vi "BeginTest.vi"(8 "error in":errorcluster) -> (0 "error out":errorcluster)   [LabVIEW 2015]
doc: "Called before other user functions, this VI is expected to open initial I/O refnums, load in file data, and do all program initialization. Notice that the <B>error out</B> terminal is simply used for data flow. Wiring it to other structures or subVIs ensures that this VI runs first."
uses:
  <vilib>/Rock Robotics/WPI/DriverStation/WPI_DriverStationRobotMode2.ctl
  <vilib>/Rock Robotics/WPI/Joystick/WPI_JoystickDeviceEnum.ctl
  <vilib>/Rock Robotics/WPI/Solenoid/WPI_SolenoidChannel.ctl
  <vilib>/Rock Robotics/SystemInterfaces/DIO/FPGA_DIOChannel.ctl
  Robot Global Data.vi
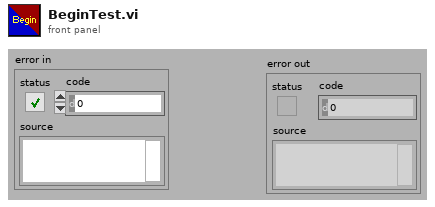
[diagram p1: front panel]
types:
  T1 = typedef "WPI_SolenoidChannel.ctl" = enum8{"Solenoid 0", "Solenoid 1", "Solenoid 2", "Solenoid 3", "Solenoid 4", "Solenoid 5", "Solenoid 6", "Solenoid 7", "Invalid"}
  T2 = typedef "FPGA_DIOChannel.ctl" = enum8{"DIO 0", "DIO 1", "DIO 2", "DIO 3", "DIO 4", "DIO 5", "DIO 6", "DIO 7", "DIO 8", "DIO 9", "DIO MXP 0", "DIO MXP 1", "DIO MXP 2", "DIO MXP 3", "DIO MXP 4", "DIO MXP 5", "DIO MXP 6", "DIO MXP 7", "DIO MXP 8", "DIO MXP 9", "DIO MXP 10", "DIO MXP 11", "DIO MXP 12", "DIO MXP 13", "DIO MXP 14", "DIO MXP 15", "Invalid"}
  T3 = cluster{"PushSolenoid":T1, "AngleMotor":cluster{"AngleMotor#":u8, "Invert AngleMotor?":bool, "PotScale":u32}, "Wheels":cluster{"LeftWheel#":u8, "Invert LeftWheel?":bool, "RightWheel#":u8, "Invert RightWheel?":bool, "WheelEncoderScale":u32}, "AnglePID":cluster{dbl, dbl, dbl}, "WheelPID":cluster{dbl, dbl, dbl}, "TopHallDIO":T2, "BottomHallDIO":T2}
  T4 = typedef "WPI_JoystickDeviceEnum.ctl" = enum16{"USB 0", "USB 1", "USB 2", "USB 3", "USB 4", "USB 5"}
  T5 = typedef "WPI_DriverStationRobotMode2.ctl" = enum16{"Autonomous Disabled", "Autonomous Enabled", "Teleop Disabled", "Teleop Enabled", "Disconnected", "Finish", "Test Disabled", "Test Enabled", "Emergency Stopped"}
  T6 = typedef "WPI_JoystickDevRef.ctl" = cluster{"Device":T4}
  T7 = typedef "WPI_SerialPortRef.ctl" = cluster{"DevStatus":errorcluster, "Serial Port Name":refnum<visa-resource-name>}
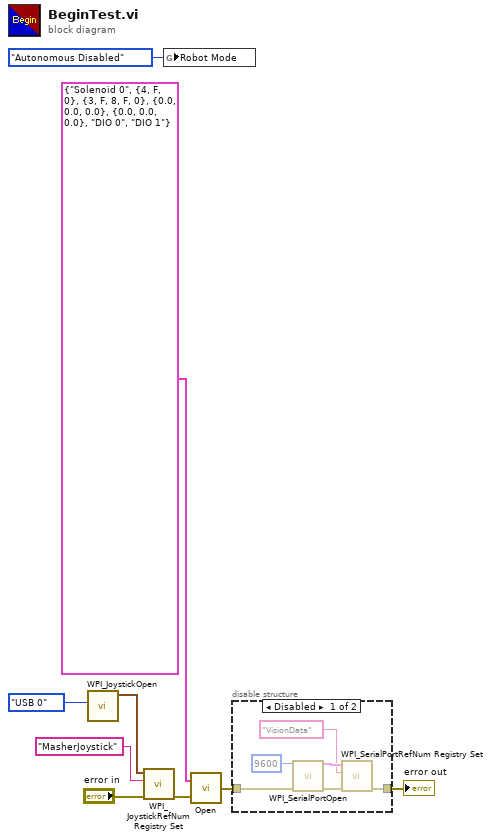
[diagram p0: block diagram]
diagram:
  n1 = call <vilib>:"WPI_JoystickOpen.vi"("JoystickDevice"=WPI_JoystickDeviceEnum."USB 0") -> ("JoystickDevRef"=w7:T6)  [unwired: 10 in]
  n2 = call <vilib>:"WPI_JoystickRefNum Registry Set.vi"("error in (no error)"="error in", "refnum name"="MasherJoystick", "JoystickDevRef"=w7) -> ("error out"=w4:errorcluster)  [unwired: 7 in, 1 out]
  n3 = global write "Robot Global Data.vi" "Robot Mode"(WPI_DriverStationRobotMode2."Autonomous Disabled" ("Robot Mode")) -> ()
  n4 = call "Open.vi"("error in"=w4, "input cluster"=T3 {"PushSolenoid"=enum."Solenoid 0", "AngleMotor"={"AngleMotor#"=4, "Invert AngleMotor?"=FALSE, "PotScale"=0}, "Wheels"={"LeftWheel#"=3, "Invert LeftWheel?"=FALSE, "RightWheel#"=8, "Invert RightWheel?"=FALSE, "WheelEncoderScale"=0}, "AnglePID"={0.0, 0.0, 0.0}, "WheelPID"={0.0, 0.0, 0.0}, "TopHallDIO"=enum."DIO 0", "BottomHallDIO"=enum."DIO 1"}) -> ("error out"=w2:errorcluster)
  n5 = disable-structure shown="Disabled" {
    disable-tunnel: w2 -> [w11 _]
    disable-tunnel: [w10 _] -> w1
    frame Disabled {
      n6 = call <vilib>:"WPI_SerialPortOpen.vi"("Baud Rate"=u32 9600, "error in (no error)"=w11) -> ("SerialPortRef"=w13:T7, "error out"=w14:errorcluster)  [unwired: 12 in]
      n7 = call <vilib>:"WPI_SerialPortRefNum Registry Set.vi"("error in (no error)"=w14, "refnum name"="VisionData", "SerialPortRef"=w13) -> ("error out"=w10:errorcluster)  [unwired: 7 in, 1 out]
    }
    frame Enabled {
    }
  }
  "error out" <- w1
